vi "Debug Interface.vi"() -> ()   [LabVIEW 2014, in "Motor manager.lvlib"]
uses:
  Motor manager.lvlib
  <vilib>/Instr/_visa.llb/VISA Configure Serial Port (Instr).vi
  Typedef/Motor.ctl
  Typedef/Move type.ctl
  Typedef/Motor settings.ctl
panel:
  out "Return":u32
  in  "Motor index":u8
  in  "Command type":T1(ring)
  in  "Write":bool
  in  "Motor settings array":T2[](array[typedef]) {"N cycles" step=1; "IM Idle time" format="%#_gms"; "Travel distance" format="%#_gmm"; "Speed" format="%#_gmm/s"}
  out "Read Buffer (Byte format)":u8[](array[numeric])
  in  "Exit":bool
  out "Bytes to read":u32
  out "Read Buffer (String format)":string
  in  "VISA in":refnum<visa-resource-name>
  # "Write"
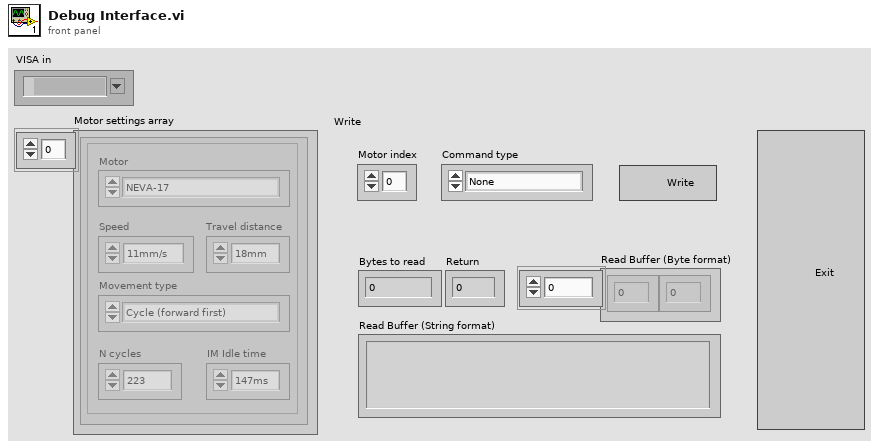
[diagram p1: front panel]
types:
  T1 = enum16{"None", "Set Motor", "Set Distance", "Set Speed", "Set Move Type", "Set IM time", "Set NCycles", "Start", "Stop"}
  T2 = typedef "Motor manager.lvlib/Motor settings.ctl" = cluster{"Motor":T3, "Speed":sgl, "Travel distance":sgl, "Movement type":T4, "IM Idle time":u32, "N cycles":u32}
  T3 = typedef "Motor manager.lvlib/Motor.ctl" = enum16{"NEVA-17"}
  T4 = typedef "Motor manager.lvlib/Move type.ctl" = enum16{"Move forward", "Move backward", "Cycle (forward first)", "Cycle (backward first)"}
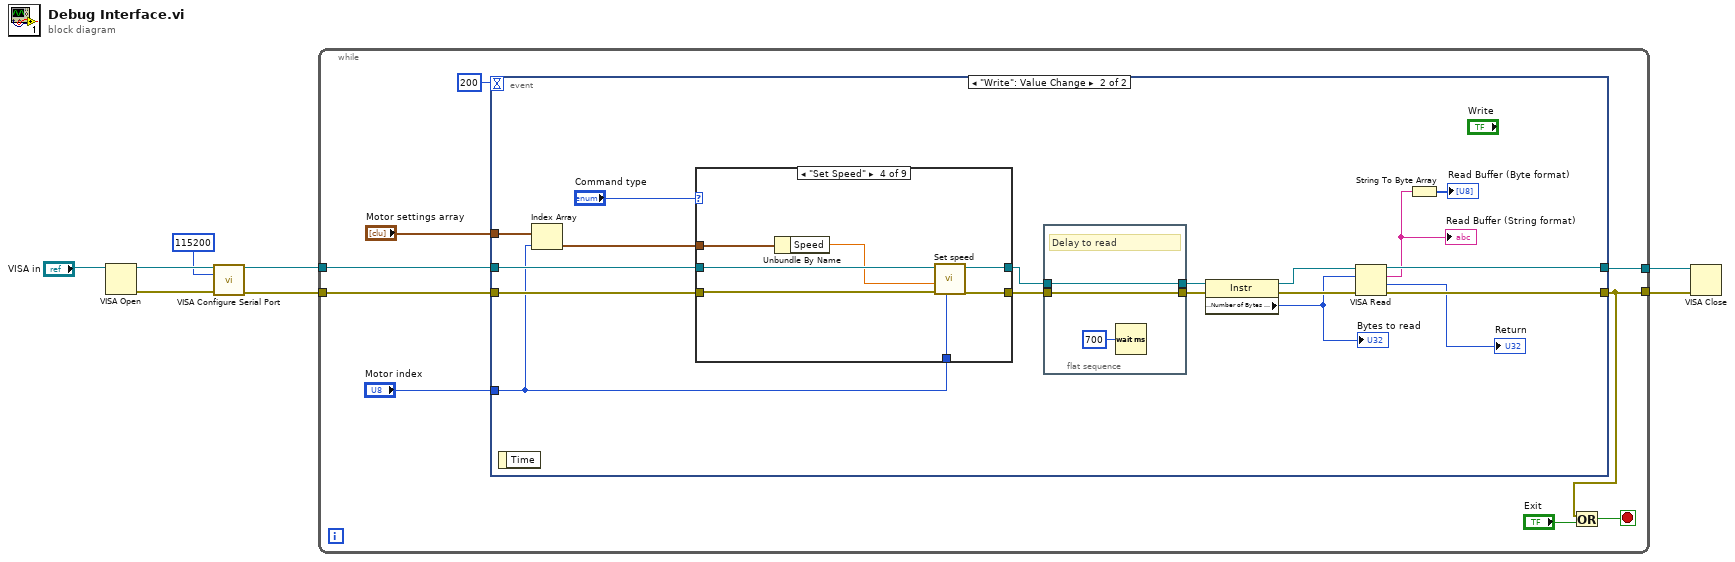
[diagram p0: block diagram]
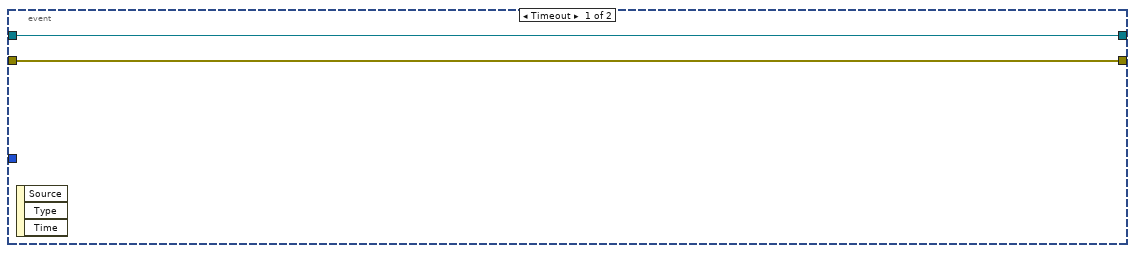
[diagram p2: hidden frame]
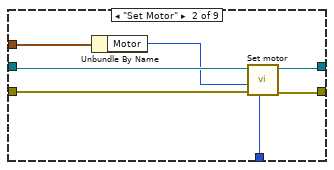
[diagram p4: hidden frame]
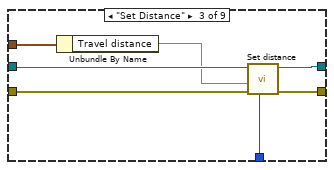
[diagram p5: hidden frame]
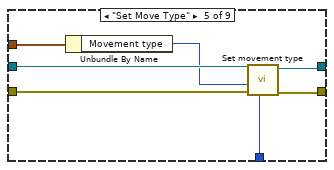
[diagram p6: hidden frame]
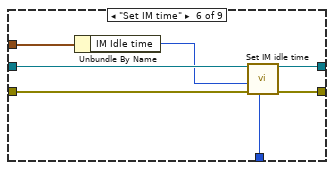
[diagram p7: hidden frame]
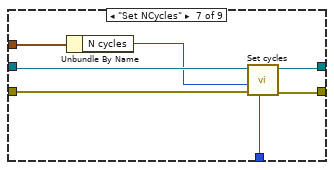
[diagram p8: hidden frame]
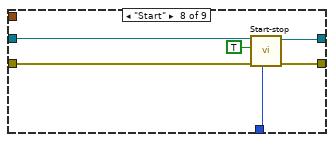
[diagram p9: hidden frame]
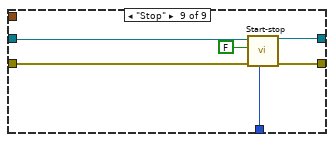
[diagram p10: hidden frame]
diagram:
  n1 = VISA Open(VISA resource name="VISA in") -> (VISA resource name=w5:refnum<visa-resource-name>, error out=w4:errorcluster)  [unwired: 4 in]
  n2 = call-poly "VISA Configure Serial Port"("VISA resource name"=w5, "baud rate (9600)"=u32 115200, "error in (no error)"=w4) -> ("VISA resource name out"=w2:refnum<visa-resource-name>, "error out"=w1:errorcluster)  [unwired: 11 in]
  n3 = while {
    tunnel: w2 -> [w15]
    tunnel: w1 -> [w14]
    tunnel: [w13] -> w8
    tunnel: [w12] -> w7
    stop <- w17 stop-if-true
    n4 = event shown="[1] \"Write\": Value Change" {
      selector: _ -> [_ _]
      dyn-events: _ -> [_ _]
      timeout: 200 -> [_ _]
      tunnel: w15 -> [w19 w37]
      tunnel: w14 -> [w18 w36]
      tunnel: "Motor settings array" -> [_ w23]
      tunnel: [w19 w30] -> w12
      tunnel: [w18 w31] -> w13
      tunnel: "Motor index" -> [_ w22]
      event Timeout {
        n5 = event-data() -> ()  [unwired: 1 in, 3 out]
      }
      event "Write": Value Change {
        n6 = event-data() -> ()  [unwired: 1 in, 1 out]
        n7 = Index Array(array=w23, index=w22) -> (element=w21:T2)
        n8 = case shown="\"Set Speed\"" "Command type" {
          tunnel: w37 -> [w42 w48 w53 w63 w70 w77 w84 w87 w92]
          tunnel: w36 -> [w41 w49 w56 w60 w69 w76 w83 w90 w93]
          tunnel: [w42 w47 w54 w62 w67 w74 w81 w88 w95] -> w25
          tunnel: [w41 w46 w55 w61 w68 w75 w82 w89 w94] -> w26
          tunnel: w22 -> [_ w45 w52 w59 w66 w73 w80 w85 w91]
          tunnel: w21 -> [_ w44 w51 w58 w65 w72 w79 _ _]
          frame "None", Default {
          }
          frame "Set Motor" {
            n9 = Unbundle By Name(w44) -> ("Motor"=w43:T3)
            n10 = call "Set motor.vi"(6:w45, "Error In"=w49, "Motor index"=w43, "VISA resource in"=w48) -> ("Error Out"=w46:errorcluster, "VISA resource out"=w47:refnum<visa-resource-name>)  [unwired: 6 in]
          }
          frame "Set Distance" {
            n11 = Unbundle By Name(w51) -> ("Travel distance"=w50:sgl)
            n12 = call "Set distance.vi"(6:w52, "Error In"=w56, "Motor index"=w50, "VISA resource in"=w53) -> ("Error Out"=w55:errorcluster, "VISA resource out"=w54:refnum<visa-resource-name>)  [unwired: 6 in]
          }
          frame "Set Speed" {
            n13 = Unbundle By Name(w58) -> ("Speed"=w57:sgl)
            n14 = call "Set speed.vi"(6:w59, "Error In"=w60, "Motor index"=w57, "VISA resource in"=w63) -> ("Error Out"=w61:errorcluster, "VISA resource out"=w62:refnum<visa-resource-name>)  [unwired: 6 in]
          }
          frame "Set Move Type" {
            n15 = Unbundle By Name(w65) -> ("Movement type"=w64:T4)
            n16 = call "Set movement type.vi"(6:w66, "Error In"=w69, "Motor index"=w64, "VISA resource in"=w70) -> ("Error Out"=w68:errorcluster, "VISA resource out"=w67:refnum<visa-resource-name>)  [unwired: 6 in]
          }
          frame "Set IM time" {
            n17 = Unbundle By Name(w72) -> ("IM Idle time"=w71:u32)
            n18 = call "Set IM idle time.vi"(6:w73, "Error In"=w76, "Motor index"=w71, "VISA resource in"=w77) -> ("Error Out"=w75:errorcluster, "VISA resource out"=w74:refnum<visa-resource-name>)  [unwired: 6 in]
          }
          frame "Set NCycles" {
            n19 = Unbundle By Name(w79) -> ("N cycles"=w78:u32)
            n20 = call "Set cycles.vi"(6:w80, "Error In"=w83, "Motor index"=w78, "VISA resource in"=w84) -> ("Error Out"=w82:errorcluster, "VISA resource out"=w81:refnum<visa-resource-name>)  [unwired: 6 in]
          }
          frame "Start" {
            n21 = call "Start-stop.vi"(6:w85, "Error In"=w90, "Go"=TRUE, "VISA resource in"=w87) -> ("Error Out"=w89:errorcluster, "VISA resource out"=w88:refnum<visa-resource-name>)  [unwired: 6 in]
          }
          frame "Stop" {
            n22 = call "Start-stop.vi"(6:w91, "Error In"=w93, "Go"=FALSE, "VISA resource in"=w92) -> ("Error Out"=w94:errorcluster, "VISA resource out"=w95:refnum<visa-resource-name>)  [unwired: 6 in]
          }
        }
        n23 = flat-sequence {
          tunnel: [w40] -> w27
          tunnel: w26 -> [w40]
          tunnel: w25 -> [w39]
          tunnel: [w39] -> w24
          frame #0 {
            # "Delay to read"
            n24 = Wait (ms)(milliseconds to wait=u32 700) -> ()  [unwired: 1 out]
          }
        }
        n25 = property class="Instr"(reference=w24, error in=w27) -> (reference out=w34:refnum<visa-resource-name>, error out=w33:errorcluster, "Serial Settings:Number of Bytes at Serial Port"=w32:u32)
        "Bytes to read" <- w32
        n26 = VISA Read(VISA resource name=w34, byte count=w32, error in (no error)=w33) -> (VISA resource name out=w30:refnum<visa-resource-name>, read buffer=w29:string, return count=→"Return":u32, error out=w31:errorcluster)
        "Read Buffer (String format)" <- w29
        n27 = String To Byte Array(string=w29) -> (unsigned byte array=→"Read Buffer (Byte format)":u8[])
      }
    }
    n28 = Or(x=w13, y="Exit") -> (x .or. y?=w17:bool)
  }
  n29 = VISA Close(VISA resource name=w7, error in (no error)=w8) -> ()  [unwired: 1 out]
